vi "INI.GetSpec.vi"(8 "error in (no error)":errorcluster caption="错误输入（无错误）", 9 "Specification_In":string[][](table), 10 "Spec_name":string, 11 "INI_File":path) -> (0 "error out":errorcluster, 2 "Spec":T1, 3 "ok?":bool)   [LabVIEW 2012, in "Lib_UEL.ATE.lvlib" / "Lib_App.lvlib"]
uses:
  <vilib>/Utility/config.llb/Read Key (String).vi
  Lib_App.lvlib
  <vilib>/Utility/config.llb/NI_LVConfig.lvlib
panel:
  # "说明:\n- 从配置文件读取或表格, 根据规格名称, 读取对应规格.\n- 优先从表格读取."
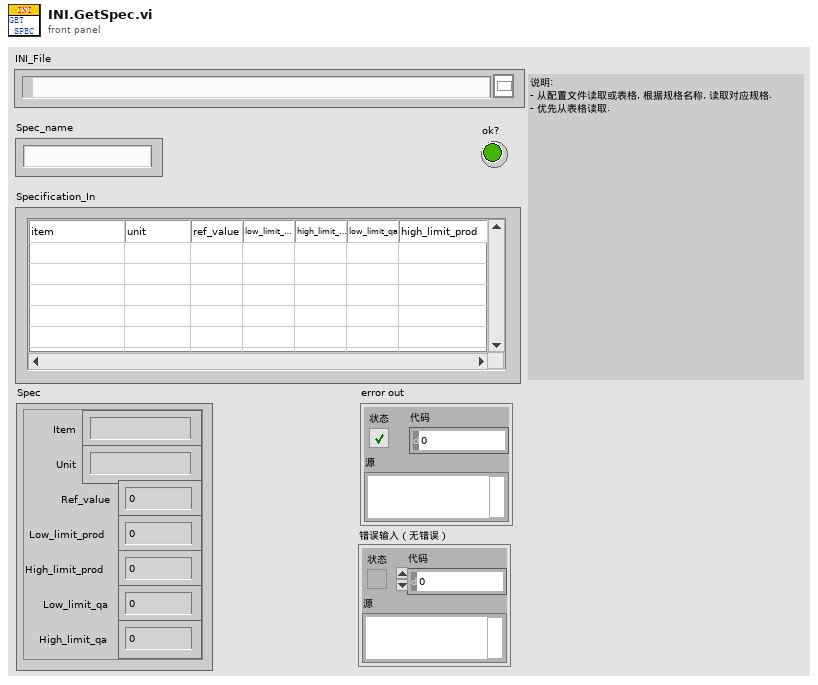
[diagram p1: front panel]
types:
  T1 = cluster{"Item":string, "Unit":string, "Ref_value":dbl, "Low_limit_prod":dbl, "High_limit_prod":dbl, "Low_limit_qa":dbl, "High_limit_qa":dbl}
  T2 = typedef "NI_LVConfig.lvlib/Config Data RefNum.ctl" = refnum<k1>
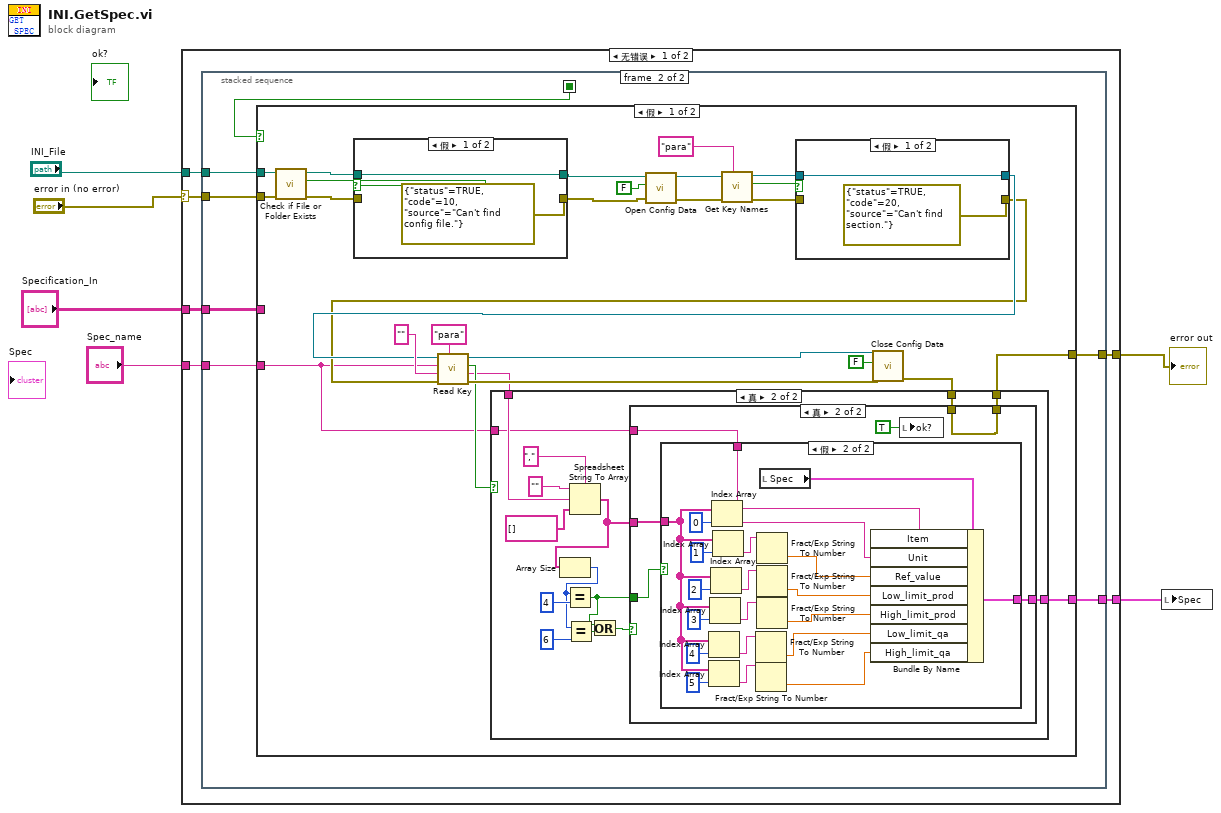
[diagram p0: block diagram]
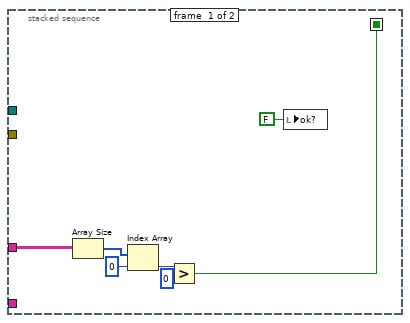
[diagram p2: hidden frame]
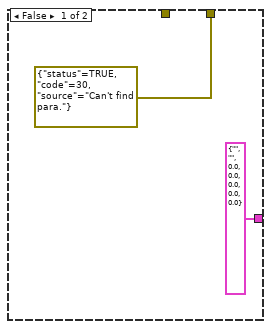
[diagram p3: hidden frame]
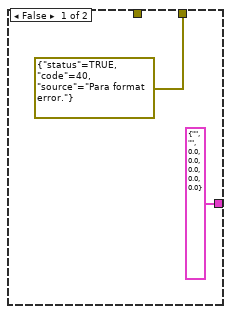
[diagram p4: hidden frame]
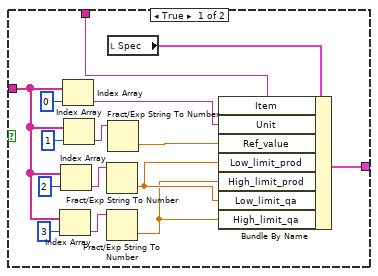
[diagram p5: hidden frame]
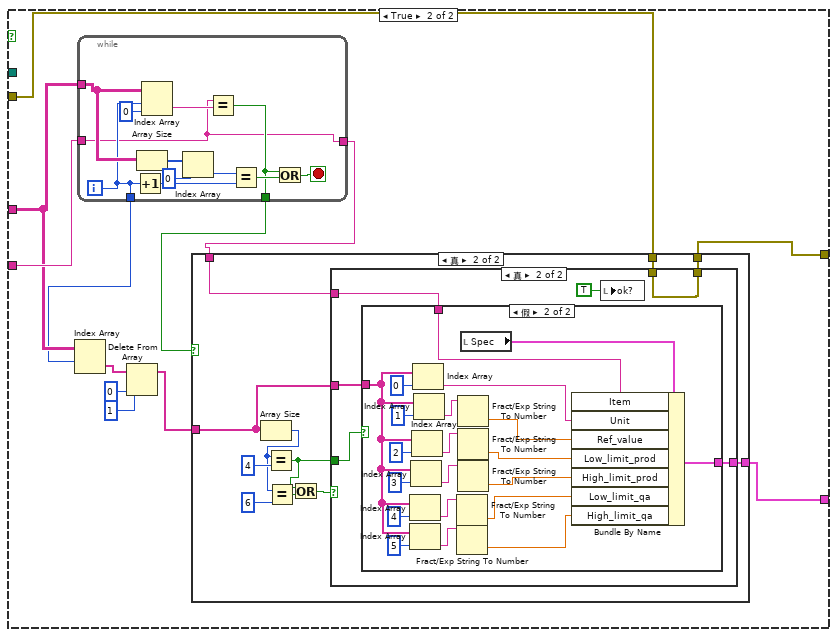
[diagram p8: hidden frame]
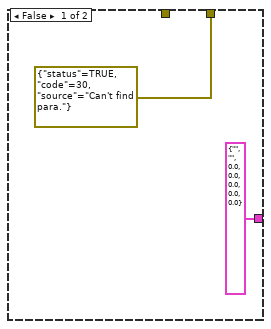
[diagram p9: hidden frame]
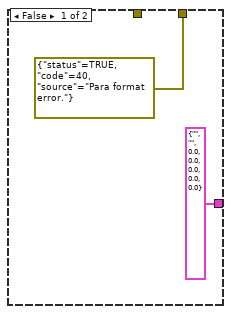
[diagram p10: hidden frame]
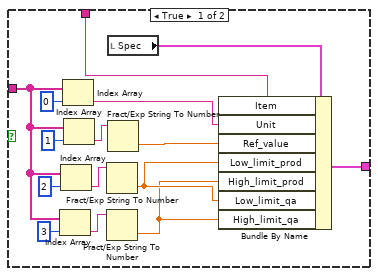
[diagram p11: hidden frame]
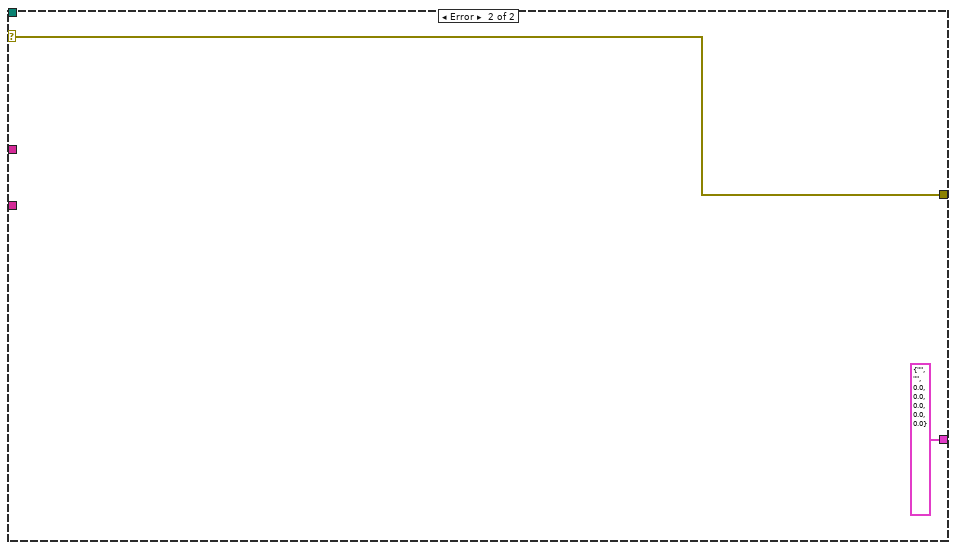
[diagram p12: hidden frame]
diagram:
  n1 = case shown="无错误" "error in (no error)" {
    selector: "error in (no error)" -> [w11 w205]
    tunnel: "INI_File" -> [w12 _]
    tunnel: [w10 w205] -> w4
    tunnel: "Specification_In" -> [w9 _]
    tunnel: "Spec_name" -> [w8 _]
    tunnel: [w7 T1 {"Item"="", "Unit"="", "Ref_value"=0.0, "Low_limit_prod"=0.0, "High_limit_prod"=0.0, "Low_limit_qa"=0.0, "High_limit_qa"=0.0} ("Spec")] -> w1
    frame No Error {
      n2 = stacked-sequence {
        seq-local: [w13 _] -> [_ w24]
        tunnel: w12 -> [_ w26]
        tunnel: w11 -> [_ w25]
        tunnel: [_ w22] -> w10
        tunnel: w9 -> [w18 w20]
        tunnel: w8 -> [_ w23]
        tunnel: [_ w21] -> w7
        frame #0 {
          n3 = Array Size(array=w18) -> (size(s)=w17:i32[])
          n4 = Index Array(array=w17, index=0 ("索引")) -> (element=w15:i32)
          n5 = Greater?(x=w15, y=0) -> (0:w13:bool)
          n6 = local write "ok?"(FALSE ("ok?")) -> ()
        }
        frame #1 {
          n7 = case shown="假" w24 {
            tunnel: w26 -> [w49 _]
            tunnel: w25 -> [w48 w131]
            tunnel: w23 -> [w27 w134]
            tunnel: [w28 w130] -> w22
            tunnel: [w30 w129] -> w21
            tunnel: w20 -> [_ w128]
            frame False {
              n8 = call <vilib>:"Check if File or Folder Exists.vi"("error in (no error)"=w48, "path"=w49) -> ("error out"=w51:errorcluster, "file or folder exists?"=w52:bool, "dup path"=w50:path)  [unwired: 7 in]
              n9 = case shown="假" w52 {
                tunnel: w51 -> [_ w121]
                tunnel: w50 -> [w120 w122]
                tunnel: [w120 w122] -> w47
                tunnel: [errorcluster {"status"=TRUE, "code"=10, "source"="Can't find config file."} ("error out") w121] -> w46
                frame False {
                }
                frame True {
                }
              }
              n10 = call <vilib>:"Open Config Data.vi"("error in (no error)"=w46, "create file if necessary (T)"=FALSE ("create file if necessary? (T)"), "configuration file path"=w47) -> ("error out"=w44:errorcluster, "refnum"=w43:T2)  [unwired: 6 in, 1 out]
              n11 = call <vilib>:"Get Key Names.vi"("section"="para", "error in (no error)"=w44, "refnum"=w43) -> ("error out"=w40:errorcluster, "section exists?"=w42:bool, "refnum out"=w41:T2)  [unwired: 5 in, 1 out]
              n12 = case shown="假" w42 {
                tunnel: w40 -> [_ w117]
                tunnel: w41 -> [w116 w118]
                tunnel: [w116 w118] -> w34
                tunnel: [errorcluster {"status"=TRUE, "code"=20, "source"="Can't find section."} ("error out") w117] -> w33
                frame False {
                }
                frame True {
                }
              }
              n13 = call-poly <vilib>:"Read Key.vi"("section"="para", "error in (no error)"=w33, "default value"="" ("section"), "key"=w27, "refnum"=w34) -> ("error out"=w37:errorcluster, "value"=w31:string, "found?"=w32:bool, "refnum out"=w38:T2)  [unwired: 3 in]
              n14 = call <vilib>:"Close Config Data.vi"("error in (no error)"=w37, "write file if changed (T)"=FALSE, "refnum"=w38) -> ("error out"=w29:errorcluster)  [unwired: 7 in, 1 out]
              n15 = case shown="真" w32 {
                tunnel: w31 -> [_ w62]
                tunnel: [T1 {"Item"="", "Unit"="", "Ref_value"=0.0, "Low_limit_prod"=0.0, "High_limit_prod"=0.0, "Low_limit_qa"=0.0, "High_limit_qa"=0.0} ("Spec") w59] -> w30
                tunnel: w29 -> [_ w58]
                tunnel: [errorcluster {"status"=TRUE, "code"=30, "source"="Can't find para."} ("error out") w57] -> w28
                tunnel: w27 -> [_ w56]
                frame False {
                }
                frame True {
                  n16 = Spreadsheet String To Array(delimiter (Tab)="," ("分隔符(Tab)"), format string="" ("格式字符串"), spreadsheet string=w62, array type (2D Dbl)=string[] [] ("数组")) -> (array=w61:string[])
                  n17 = Array Size(array=w61) -> (size(s)=w66:i32)
                  n18 = Equal?(x=w66, y=4) -> (x = y?=w60:bool)
                  n19 = Equal?(x=w66, y=6) -> (x = y?=w64:bool)
                  n20 = Or(x=w60, y=w64) -> (x .or. y?=w63:bool)
                  n21 = case shown="真" w63 {
                    tunnel: w56 -> [_ w78]
                    tunnel: w61 -> [_ w77]
                    tunnel: w60 -> [_ w76]
                    tunnel: [T1 {"Item"="", "Unit"="", "Ref_value"=0.0, "Low_limit_prod"=0.0, "High_limit_prod"=0.0, "Low_limit_qa"=0.0, "High_limit_qa"=0.0} ("Spec") w75] -> w59
                    tunnel: w58 -> [_ w74]
                    tunnel: [errorcluster {"status"=TRUE, "code"=40, "source"="Para format error."} ("error out") w74] -> w57
                    frame False {
                    }
                    frame True {
                      n22 = case shown="假" w76 {
                        tunnel: w78 -> [w92 w113]
                        tunnel: w77 -> [w85 w96]
                        tunnel: [w79 w101] -> w75
                        frame True {
                          n23 = Index Array(array=w85, index=3 ("索引")) -> (element=w82:string)
                          n24 = Index Array(array=w85, index=2 ("索引")) -> (element=w86:string)
                          n25 = Index Array(array=w85, index=0 ("索引")) -> (element=w90:string)
                          n26 = Index Array(array=w85, index=1 ("索引")) -> (element=w88:string)
                          n27 = Fract/Exp String To Number(string=w86) -> (number=w81:dbl)  [unwired: 3 in, 1 out]
                          n28 = Fract/Exp String To Number(string=w82) -> (number=w80:dbl)  [unwired: 3 in, 1 out]
                          n29 = local read "Spec"() -> (w93:T1)
                          n30 = Fract/Exp String To Number(string=w88) -> (number=w87:dbl)  [unwired: 3 in, 1 out]
                          n31 = Bundle By Name(cluster=w93, "Item"=w92, "Unit"=w90, "Ref_value"=w87, "Low_limit_prod"=w81, "High_limit_prod"=w80, "Low_limit_qa"=w81, "High_limit_qa"=w80) -> (w79:T1)
                        }
                        frame False {
                          n32 = Index Array(array=w96, index=4 ("索引")) -> (element=w100:string)
                          n33 = Index Array(array=w96, index=5 ("索引")) -> (element=w97:string)
                          n34 = Index Array(array=w96, index=3 ("索引")) -> (element=w104:string)
                          n35 = Index Array(array=w96, index=2 ("索引")) -> (element=w107:string)
                          n36 = Index Array(array=w96, index=0 ("索引")) -> (element=w111:string)
                          n37 = Index Array(array=w96, index=1 ("索引")) -> (element=w109:string)
                          n38 = Fract/Exp String To Number(string=w100) -> (number=w95:dbl)  [unwired: 3 in, 1 out]
                          n39 = Fract/Exp String To Number(string=w97) -> (number=w94:dbl)  [unwired: 3 in, 1 out]
                          n40 = Fract/Exp String To Number(string=w109) -> (number=w108:dbl)  [unwired: 3 in, 1 out]
                          n41 = Fract/Exp String To Number(string=w107) -> (number=w103:dbl)  [unwired: 3 in, 1 out]
                          n42 = Fract/Exp String To Number(string=w104) -> (number=w102:dbl)  [unwired: 3 in, 1 out]
                          n43 = local read "Spec"() -> (w114:T1)
                          n44 = Bundle By Name(cluster=w114, "Item"=w113, "Unit"=w111, "Ref_value"=w108, "Low_limit_prod"=w103, "High_limit_prod"=w102, "Low_limit_qa"=w95, "High_limit_qa"=w94) -> (w101:T1)
                        }
                      }
                      n45 = local write "ok?"(TRUE ("ok?")) -> ()
                    }
                  }
                }
              }
            }
            frame True {
              n46 = while {
                tunnel: w128 -> [w201]
                tunnel: w134 -> [w192]
                tunnel: [w195] -> w133
                tunnel: [w192] -> w132
                tunnel: [w193] -> w127
                i -> [w193]
                stop <- w202 stop-if-true
                n47 = Increment(x=w193) -> (x+1=w200:i32)
                n48 = Array Size(array=w201) -> (size(s)=w199:i32[])
                n49 = Index Array(array=w201, index (row)=w193, index (col)=0 ("禁用的索引 (列)")) -> (element=w194:string)
                n50 = Index Array(array=w199, index=0 ("索引")) -> (element=w197:i32)
                n51 = Equal?(x=w192, y=w194) -> (x = y?=w195:bool)
                n52 = Equal?(x=w197, y=w200) -> (x = y?=w196:bool)
                n53 = Or(x=w195, y=w196) -> (x .or. y?=w202:bool)
              }
              n54 = Index Array(array=w128, index (row)=w127) -> (element=w126:string[])  [unwired: 1 in]
              n55 = Delete From Array(array=w126, length=1 ("长度"), index=0 ("索引")) -> (array with subset deleted=w123:string[])  [unwired: 1 out]
              n56 = case shown="真" w133 {
                tunnel: w132 -> [_ w142]
                tunnel: [T1 {"Item"="", "Unit"="", "Ref_value"=0.0, "Low_limit_prod"=0.0, "High_limit_prod"=0.0, "Low_limit_qa"=0.0, "High_limit_qa"=0.0} ("Spec") w140] -> w129
                tunnel: w131 -> [_ w139]
                tunnel: [errorcluster {"status"=TRUE, "code"=30, "source"="Can't find para."} ("error out") w138] -> w130
                tunnel: w123 -> [_ w137]
                frame False {
                }
                frame True {
                  n57 = Array Size(array=w137) -> (size(s)=w146:i32)
                  n58 = Equal?(x=w146, y=4) -> (x = y?=w141:bool)
                  n59 = Equal?(x=w146, y=6) -> (x = y?=w144:bool)
                  n60 = Or(x=w141, y=w144) -> (x .or. y?=w143:bool)
                  n61 = case shown="真" w143 {
                    tunnel: w142 -> [_ w155]
                    tunnel: w137 -> [_ w154]
                    tunnel: w141 -> [_ w153]
                    tunnel: [T1 {"Item"="", "Unit"="", "Ref_value"=0.0, "Low_limit_prod"=0.0, "High_limit_prod"=0.0, "Low_limit_qa"=0.0, "High_limit_qa"=0.0} ("Spec") w152] -> w140
                    tunnel: w139 -> [_ w151]
                    tunnel: [errorcluster {"status"=TRUE, "code"=40, "source"="Para format error."} ("error out") w151] -> w138
                    frame False {
                    }
                    frame True {
                      n62 = case shown="假" w153 {
                        tunnel: w155 -> [w169 w190]
                        tunnel: w154 -> [w162 w173]
                        tunnel: [w156 w178] -> w152
                        frame True {
                          n63 = Index Array(array=w162, index=3 ("索引")) -> (element=w159:string)
                          n64 = Index Array(array=w162, index=2 ("索引")) -> (element=w163:string)
                          n65 = Index Array(array=w162, index=0 ("索引")) -> (element=w167:string)
                          n66 = Index Array(array=w162, index=1 ("索引")) -> (element=w165:string)
                          n67 = Fract/Exp String To Number(string=w163) -> (number=w158:dbl)  [unwired: 3 in, 1 out]
                          n68 = Fract/Exp String To Number(string=w159) -> (number=w157:dbl)  [unwired: 3 in, 1 out]
                          n69 = local read "Spec"() -> (w170:T1)
                          n70 = Fract/Exp String To Number(string=w165) -> (number=w164:dbl)  [unwired: 3 in, 1 out]
                          n71 = Bundle By Name(cluster=w170, "Item"=w169, "Unit"=w167, "Ref_value"=w164, "Low_limit_prod"=w158, "High_limit_prod"=w157, "Low_limit_qa"=w158, "High_limit_qa"=w157) -> (w156:T1)
                        }
                        frame False {
                          n72 = Index Array(array=w173, index=4 ("索引")) -> (element=w177:string)
                          n73 = Index Array(array=w173, index=5 ("索引")) -> (element=w174:string)
                          n74 = Index Array(array=w173, index=3 ("索引")) -> (element=w181:string)
                          n75 = Index Array(array=w173, index=2 ("索引")) -> (element=w184:string)
                          n76 = Index Array(array=w173, index=0 ("索引")) -> (element=w188:string)
                          n77 = Index Array(array=w173, index=1 ("索引")) -> (element=w186:string)
                          n78 = Fract/Exp String To Number(string=w177) -> (number=w172:dbl)  [unwired: 3 in, 1 out]
                          n79 = Fract/Exp String To Number(string=w174) -> (number=w171:dbl)  [unwired: 3 in, 1 out]
                          n80 = Fract/Exp String To Number(string=w186) -> (number=w185:dbl)  [unwired: 3 in, 1 out]
                          n81 = Fract/Exp String To Number(string=w184) -> (number=w180:dbl)  [unwired: 3 in, 1 out]
                          n82 = Fract/Exp String To Number(string=w181) -> (number=w179:dbl)  [unwired: 3 in, 1 out]
                          n83 = local read "Spec"() -> (w191:T1)
                          n84 = Bundle By Name(cluster=w191, "Item"=w190, "Unit"=w188, "Ref_value"=w185, "Low_limit_prod"=w180, "High_limit_prod"=w179, "Low_limit_qa"=w172, "High_limit_qa"=w171) -> (w178:T1)
                        }
                      }
                      n85 = local write "ok?"(TRUE ("ok?")) -> ()
                    }
                  }
                }
              }
            }
          }
        }
      }
    }
    frame Error {
    }
  }
  "error out" <- w4
  n86 = local write "Spec"(w1) -> ()
